vi "ReverseDrive.vi"() -> ()   [LabVIEW 2012]
panel:
  in  "Backup speed":dbl
  out "Starboard Speed":i32(knob) scale=1000.0..2000.0
  out "Port Speed":i32(knob) scale=1000.0..2000.0
  out "Elapsed Time (s)":dbl
  out "Finished running":bool
  in  "Backup time (s)":dbl
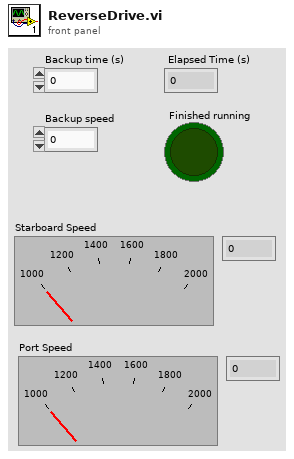
[diagram p1: front panel]
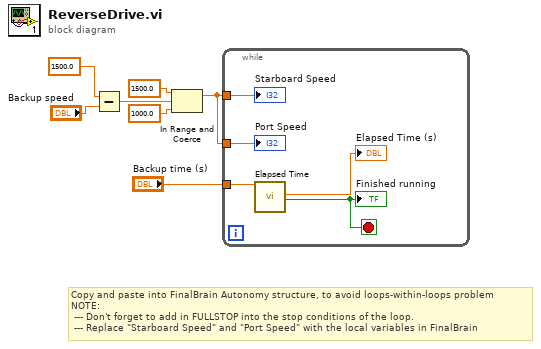
[diagram p0: block diagram]
diagram:
  # "Copy and paste into FinalBrain Autonomy structure, to avoid loops-within-loops problem\nNOTE: \n --- Don't forget to add in FULLSTOP into the stop conditions of the loop. \n --- Replace \"Starboard Speed\" and \"Port Speed\" with the local variables in FinalBrain"
  n1 = Subtract(x=1500.0, y="Backup speed") -> (x-y=w1:dbl)
  n2 = In Range and Coerce(upper limit=1500.0, x=w1, lower limit=1000.0) -> (coerced(x)=w4:dbl)  [unwired: 1 out]
  n3 = while {
    tunnel: "Backup time (s)" -> [w12]
    tunnel: w4 -> [w9]
    tunnel: w4 -> [w8]
    stop <- w11 stop-if-true
    n4 = call "Elapsed Time"("Time Target (s)"=w12) -> ("Elapsed Time (s)"=→"Elapsed Time (s)":dbl, "Time has Elapsed"=w11:bool)  [unwired: 11 in, 6 out]
    "Finished running" <- w11
    "Port Speed" <- w8
    "Starboard Speed" <- w9
  }
